vi "Configure Imaqdx.vi"(8 "error in":errorcluster, 11 "IMAQdx Base Configure Strategy in":refnum<class "IMAQdx Base Configure Strategy.lvclass">) -> (0 "error out":errorcluster, 3 "IMAQdx Base Configure Strategy out":refnum<class "IMAQdx Base Configure Strategy.lvclass">)   [LabVIEW 2024, in "IMAQdx Base Configure Strategy.lvclass"]
uses:
  IMAQdx Base Configure Strategy.lvclass
  IMAQdx Base Configure Strategy.lvclass/IMAQdx Base Configure Strategy.ctl
  Source/Interfaces/IConfiguration/IConfiguration.lvclass
  Source/Typedefs/Generic Image/Pixel Format.ctl
  Source/Typedefs/Generic Image/Generic Image.lvclass
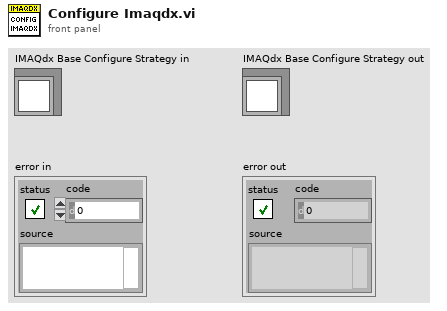
[diagram p1: front panel]
types:
  T1 = typedef "Generic Image.lvclass/Pixel Format.ctl" = enum16{"Grayscale (U8)", "Grayscale (I16)", "Grayscale (SGL)", "Complex (CSG)", "RGB (U32)", "HSL (U32)", "RGB (U64)", "Grayscale (U16)"}
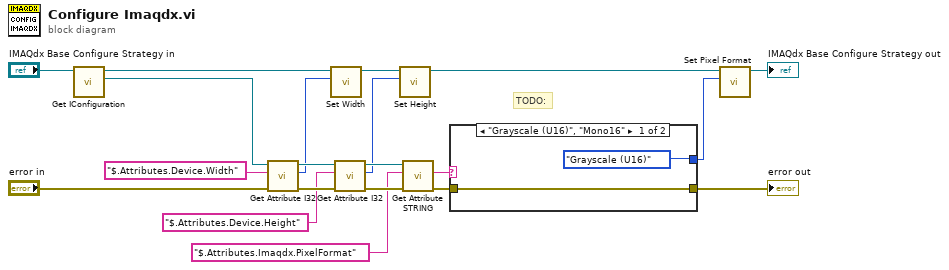
[diagram p0: block diagram]
diagram:
  # "TODO:"
  n1 = call-dynamic "Get IConfiguration.vi"("IMAQdx Base Configure Strategy in"="IMAQdx Base Configure Strategy in") -> ("IConfiguration"=w10:refnum<class "IConfiguration.lvclass">, "IMAQdx Base Configure Strategy out"=w11:refnum<class "IMAQdx Base Configure Strategy.lvclass">)  [unwired: 9 in]
  n2 = call-dynamic "Get Attribute I32.vi"("error in"="error in", "Attribute"="$.Attributes.Device.Width", "IConfiguration in"=w10) -> ("error out"=w19:errorcluster, "Value"=w6:i32, "IConfiguration out"=w16:refnum<class "IConfiguration.lvclass">)  [unwired: 6 in]
  n3 = call "Set Width.vi"("Width"=w6, "IMAQdx Base Configure Strategy in"=w11) -> ("IMAQdx Base Configure Strategy out"=w9:refnum<class "IMAQdx Base Configure Strategy.lvclass">)  [unwired: 9 in]
  n4 = call-dynamic "Get Attribute I32.vi"("error in"=w19, "Attribute"="$.Attributes.Device.Height", "IConfiguration in"=w16) -> ("error out"=w17:errorcluster, "Value"=w5:i32, "IConfiguration out"=w14:refnum<class "IConfiguration.lvclass">)  [unwired: 6 in]
  n5 = call "Set Height.vi"("Height"=w5, "IMAQdx Base Configure Strategy in"=w9) -> ("IMAQdx Base Configure Strategy out"=w8:refnum<class "IMAQdx Base Configure Strategy.lvclass">)  [unwired: 9 in]
  n6 = call-dynamic "Get Attribute STRING.vi"("error in"=w17, "Attribute"="$.Attributes.Imaqdx.PixelFormat", "IConfiguration in"=w14) -> ("error out"=w2:errorcluster, "Value"=w1:string)  [unwired: 6 in, 1 out]
  n7 = case shown="\"Grayscale (U16)\", \"Mono16\"" w1 {
    tunnel: [w22 w23] -> w4
    tunnel: [Pixel_Format."Grayscale (U16)" ("Image Format.Pixel Format") _] -> w3
    tunnel: w2 -> [w22 w23]
    frame "Grayscale (U16)", "Mono16" {
    }
    frame Default {
    }
  }
  "error out" <- w4
  n8 = call "Set Pixel Format.vi"("Pixel Format"=w3, "IMAQdx Base Configure Strategy in"=w8) -> ("IMAQdx Base Configure Strategy out"=→"IMAQdx Base Configure Strategy out":refnum<class "IMAQdx Base Configure Strategy.lvclass">)  [unwired: 9 in]
